vi "test_crc8.vi"() -> (3 "All Passed?":bool)   [LabVIEW 2021]
uses:
  src/hashlib.lvlib
panel:
  in  "Data in":string="123456789"
  out "CRC-8 out":T1(array[cluster]) {"CRC-8" format="%02x"}
  in  "CRC-8 Types":T2(array[cluster])=[{"Name"="CRC-8", "CRC8"=244, "Initial"=0, "Poly"=7, "XorOut"=0, "ReflectIn"=FALSE, "ReflectOut"=FALSE}, {"Name"="CRC-8/CDMA2000", "CRC8"=218, "Initial"=255, "Poly"=155, "XorOut"=0, "ReflectIn"=FALSE, "ReflectOut"=FALSE}, {"Name"="CRC-8/DARC", "CRC8"=21, "Initial"=0, "Poly"=57, "XorOut"=0, "ReflectIn"=TRUE, "ReflectOut"=TRUE}, {"Name"="CRC-8/DVB-S2", "CRC8"=188, "Initial"=0, "Poly"=213, "XorOut"=0, "ReflectIn"=FALSE, "ReflectOut"=FALSE}, {"Name"="CRC-8/EBU", "CRC8"=151, "Initial"=255, "Poly"=29, "XorOut"=0, "ReflectIn"=TRUE, "ReflectOut"=TRUE}, {"Name"="CRC-8/I-CODE", "CRC8"=126, "Initial"=253, "Poly"=29, "XorOut"=0, "ReflectIn"=FALSE, "ReflectOut"=FALSE}, {"Name"="CRC-8/ITU", "CRC8"=161, "Initial"=0, "Poly"=7, "XorOut"=85, "ReflectIn"=FALSE, "ReflectOut"=FALSE}, {"Name"="CRC-8/MAXIM", "CRC8"=161, "Initial"=0, "Poly"=49, "XorOut"=0, "ReflectIn"=TRUE, "ReflectOut"=TRUE}, {"Name"="CRC-8/ROHC", "CRC8"=208, "Initial"=255, "Poly"=7, "XorOut"=0, "ReflectIn"=TRUE, "ReflectOut"=TRUE}, {"Name"="CRC-8/WCDMA", "CRC8"=37, "Initial"=0, "Poly"=155, "XorOut"=0, "ReflectIn"=TRUE, "ReflectOut"=TRUE}] {"XorOut" format="%02x"; "CRC8" format="%02x"; "Poly" format="%02x"; "Initial" format="%02x"}
  # "https://crccalc.com/"
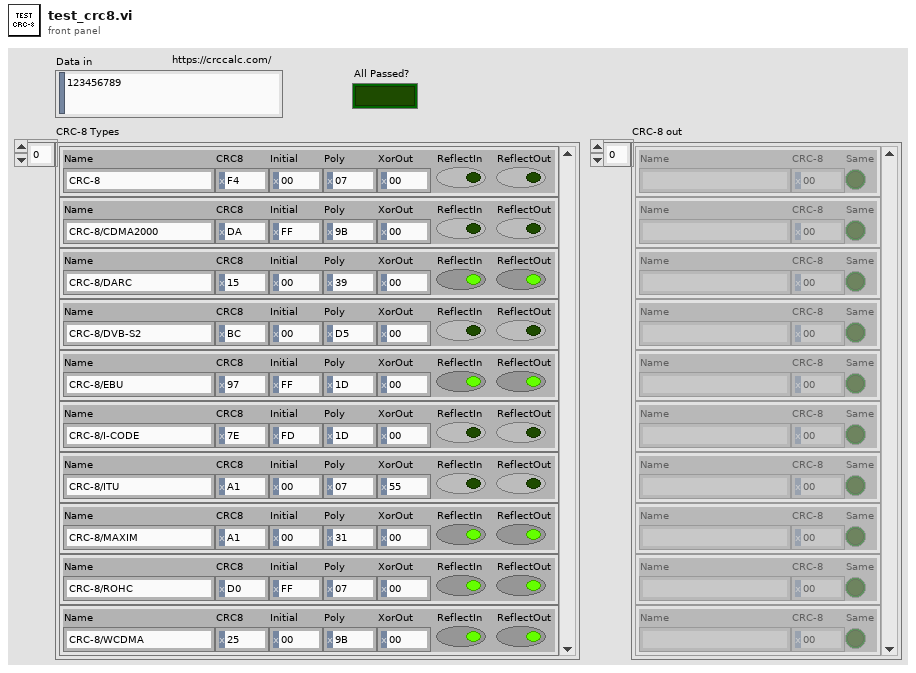
[diagram p1: front panel]
types:
  T1 = cluster{"Name":string, "CRC-8":u8, "Same":bool}[]
  T2 = cluster{"Name":string, "CRC8":u8, "Initial":u8, "Poly":u8, "XorOut":u8, "ReflectIn":bool, "ReflectOut":bool}[]
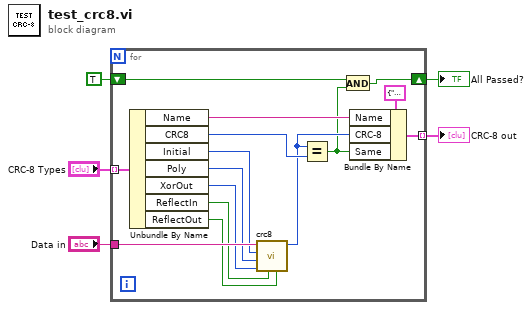
[diagram p0: block diagram]
diagram:
  n1 = for {
    tunnel: "Data in" -> [w20]
    tunnel: "CRC-8 Types" -> [w19] mode=indexing
    tunnel: [w17] -> w3 mode=indexing
    shift-right: [w12] -> w1
    shift-left: TRUE -> [w14]
    n2 = Unbundle By Name(w19) -> ("Name"=w18:string, "CRC8"=w16:u8, "Initial"=w11:u8, "Poly"=w10:u8, "XorOut"=w9:u8, "ReflectIn"=w8:bool, "ReflectOut"=w7:bool)
    n3 = call "crc8.vi"("Reflect Output? (F)"=w7, "Reflect Input? (F)"=w8, "Xor Out (0x00)"=w9, "Poly (0x07)"=w10, "Init (0x00)"=w11, "Data in"=w20) -> ("CRC-8"=w15:u8)  [unwired: 5 in]
    n4 = Equal?(x=w15, y=w16) -> (x = y?=w13:bool)
    n5 = And(x=w14, y=w13) -> (x .and. y?=w12:bool)
    n6 = Bundle By Name(cluster=cluster{"Name":string, "CRC-8":u8, "Same":bool} {"Name"="", "CRC-8"=0, "Same"=FALSE} ("CRC-16"), "Name"=w18, "CRC-8"=w15, "Same"=w13) -> (w17:cluster{"Name":string, "CRC-8":u8, "Same":bool})
  }
  "CRC-8 out" <- w3
  "All Passed?" <- w1
